vi "ke37xx Simple Switching Example.vi"() -> ()   [LabVIEW 2009]
doc: "Simple Switching Example \n\nThis sample demonstrates use of basic channel operations \nsupported by the Ke37XX. A channel list can be specified\non which various switch commands can be performed. After\neach switch operation, the current state of switch closures\nin the instrument is updated and displayed in the \"Channel \nStatus\" panel.\n\nUse of Pseudo Cards\n\nThis sample can be run using a mainframe that has no cards\npresent in the system slots (1 to 6). This is accomplished\nby use of the Ke37XX's native support for \"pseudo cards\".\nBy using pseudo cards, instrument commands may be sent to\nthe Ke37XX as if the cards were physically present. The \ninstrument responses will be simulated by the instrument itself.\nCombo boxes are provided for specifying which card should be\nsimulated in each slot."
uses:
  <instrlib>/Keithley 3706/Keithley 3700 Series.lvlib
panel:
  out "Close Channel List":string
  in  "Operation":T1(ring)
  in  "Channel List":string="1001:1005"
  in  "Slot 6 Pseudocard (6: 3740)":u16(ring)=6 items=["Empty", "3720", "3721", "3722", "3723", "3730", "3740"]
  in  "Slot 5 Pseudocard (5: 3730)":u16(ring)=5 items=["Empty", "3720", "3721", "3722", "3723", "3730", "3740"]
  in  "Slot 4 Pseudocard (4: 3723)":u16(ring)=4 items=["Empty", "3720", "3721", "3722", "3723", "3730", "3740"]
  in  "Slot 3 Pseudocard (3: 3722)":u16(ring)=3 items=["Empty", "3720", "3721", "3722", "3723", "3730", "3740"]
  in  "Slot 2 Pseudocard (2: 3721)":u16(ring)=2 items=["Empty", "3720", "3721", "3722", "3723", "3730", "3740"]
  in  "Slot 1 Pseudocard (1: 3720)":u16(ring)=1 items=["Empty", "3720", "3721", "3722", "3723", "3730", "3740"]
  in  "VISA Resource Name":refnum<visa-resource-name>="GPIB::6"
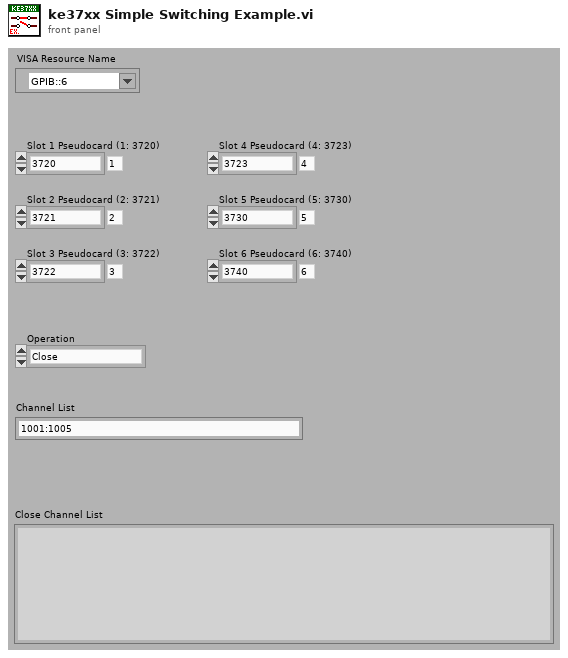
[diagram p1: front panel]
types:
  T1 = enum16{"Close", "Close Exclusive", "Close Slot Exclusive", "Open", "Open All"}
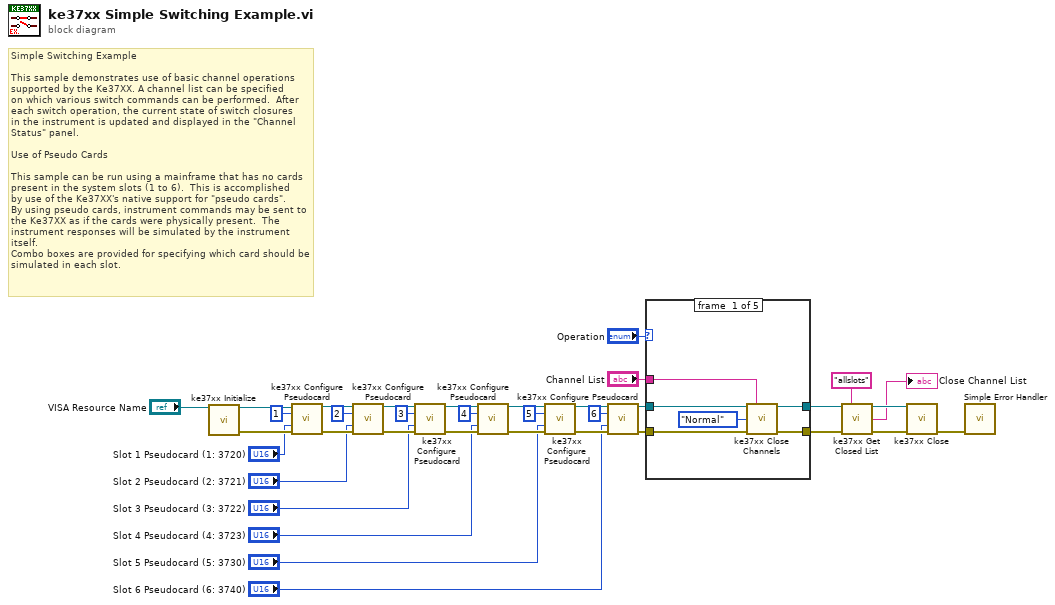
[diagram p0: block diagram]
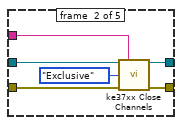
[diagram p2: hidden frame]
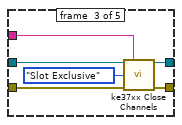
[diagram p3: hidden frame]
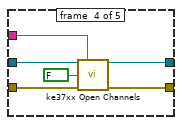
[diagram p4: hidden frame]
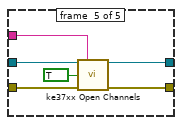
[diagram p5: hidden frame]
diagram:
  # "Simple Switching Example                              \n\nThis sample demonstrates use of basic channel operations \nsupported by the Ke37XX. A channel list can be specified\non which various switch commands can be performed.  After\neach switch operation, the current state of switch closures\nin the instrument is updated and displayed in the \"Channel \nStatus\" panel.\n\nUse of Pseudo Cards\n\nThis sample can be run using a mainframe that has no cards\npresent in the system slots (1 to 6).  This is accomplished\nby use of the Ke37XX's native support for \"pseudo cards\".\nBy using pseudo cards, instrument commands may be sent to\nthe Ke37XX as if the cards were physically present.  The \ninstrument responses will be simulated by the instrument itself.\nCombo boxes are provided for specifying which card should be\nsimulated in each slot."
  n1 = call <instrlib>:"ke37xx Initialize.vi"("VISA resource name"="VISA Resource Name") -> ("VISA resource name out"=w11:refnum<visa-resource-name>, "error out"=w36:errorcluster)  [unwired: 13 in]
  n2 = call <instrlib>:"ke37xx Configure Pseudocard.vi"("VISA Resource Name"=w11, "Slot Number (1)"=1, "Pseudocard Name (1: 3720)"="Slot 1 Pseudocard (1: 3720)", "error in (no error)"=w36) -> ("VISA Resource Name Out"=w27:refnum<visa-resource-name>, "error out"=w21:errorcluster)  [unwired: 10 in]
  n3 = call <instrlib>:"ke37xx Configure Pseudocard.vi"("VISA Resource Name"=w27, "Slot Number (1)"=2, "Pseudocard Name (1: 3720)"="Slot 2 Pseudocard (2: 3721)", "error in (no error)"=w21) -> ("VISA Resource Name Out"=w26:refnum<visa-resource-name>, "error out"=w20:errorcluster)  [unwired: 10 in]
  n4 = call <instrlib>:"ke37xx Configure Pseudocard.vi"("VISA Resource Name"=w26, "Slot Number (1)"=3, "Pseudocard Name (1: 3720)"="Slot 3 Pseudocard (3: 3722)", "error in (no error)"=w20) -> ("VISA Resource Name Out"=w25:refnum<visa-resource-name>, "error out"=w19:errorcluster)  [unwired: 10 in]
  n5 = call <instrlib>:"ke37xx Configure Pseudocard.vi"("VISA Resource Name"=w25, "Slot Number (1)"=4, "Pseudocard Name (1: 3720)"="Slot 4 Pseudocard (4: 3723)", "error in (no error)"=w19) -> ("VISA Resource Name Out"=w24:refnum<visa-resource-name>, "error out"=w18:errorcluster)  [unwired: 10 in]
  n6 = call <instrlib>:"ke37xx Configure Pseudocard.vi"("VISA Resource Name"=w24, "Slot Number (1)"=5, "Pseudocard Name (1: 3720)"="Slot 5 Pseudocard (5: 3730)", "error in (no error)"=w18) -> ("VISA Resource Name Out"=w23:refnum<visa-resource-name>, "error out"=w17:errorcluster)  [unwired: 10 in]
  n7 = call <instrlib>:"ke37xx Configure Pseudocard.vi"("VISA Resource Name"=w23, "Slot Number (1)"=6, "Pseudocard Name (1: 3720)"="Slot 6 Pseudocard (6: 3740)", "error in (no error)"=w17) -> ("VISA Resource Name Out"=w9:refnum<visa-resource-name>, "error out"=w8:errorcluster)  [unwired: 10 in]
  n8 = case shown="\"Close Slot Exclusive\"" "Operation" {
    tunnel: w9 -> [w42 w48 w54 w60 w66]
    tunnel: w8 -> [w41 w47 w53 w59 w65]
    tunnel: [w40 w46 w52 w58 w64] -> w7
    tunnel: [w39 w45 w51 w57 w63] -> w6
    tunnel: "Channel List" -> [w37 w43 w49 w56 w62]
    frame #0 {
      n9 = call <instrlib>:"ke37xx Close Channels.vi"("VISA Resource Name"=w42, "Channel List"=w37, "Mode (0: Normal)"=enum16{"Normal", "Exclusive", "Slot Exclusive"}."Normal", "error in (no error)"=w41) -> ("VISA Resource Name Out"=w40:refnum<visa-resource-name>, "error out"=w39:errorcluster)  [unwired: 10 in]
    }
    frame #1 {
      n10 = call <instrlib>:"ke37xx Close Channels.vi"("VISA Resource Name"=w48, "Channel List"=w43, "Mode (0: Normal)"=enum16{"Normal", "Exclusive", "Slot Exclusive"}."Exclusive", "error in (no error)"=w47) -> ("VISA Resource Name Out"=w46:refnum<visa-resource-name>, "error out"=w45:errorcluster)  [unwired: 10 in]
    }
    frame #2 {
      n11 = call <instrlib>:"ke37xx Close Channels.vi"("VISA Resource Name"=w54, "Channel List"=w49, "Mode (0: Normal)"=enum16{"Normal", "Exclusive", "Slot Exclusive"}."Slot Exclusive", "error in (no error)"=w53) -> ("VISA Resource Name Out"=w52:refnum<visa-resource-name>, "error out"=w51:errorcluster)  [unwired: 10 in]
    }
    frame #3 {
      n12 = call <instrlib>:"ke37xx Open Channels.vi"("VISA Resource Name"=w60, "Channel List"=w56, "Open All (False)"=FALSE, "error in (no error)"=w59) -> ("VISA Resource Name Out"=w58:refnum<visa-resource-name>, "error out"=w57:errorcluster)  [unwired: 10 in]
    }
    frame #4 {
      n13 = call <instrlib>:"ke37xx Open Channels.vi"("VISA Resource Name"=w66, "Channel List"=w62, "Open All (False)"=TRUE, "error in (no error)"=w65) -> ("VISA Resource Name Out"=w64:refnum<visa-resource-name>, "error out"=w63:errorcluster)  [unwired: 10 in]
    }
  }
  n14 = call <instrlib>:"ke37xx Get Closed List.vi"("VISA Resource Name"=w7, "Channel List"="allslots", "error in (no error)"=w6) -> ("VISA Resource Name Out"=w5:refnum<visa-resource-name>, "Closed List"=→"Close Channel List":string, "error out"=w4:errorcluster)  [unwired: 10 in]
  n15 = call <instrlib>:"ke37xx Close.vi"("VISA resource name"=w5, "error in (no error)"=w4) -> ("error out"=w34:errorcluster)  [unwired: 13 in]
  n16 = call <vilib>:"Simple Error Handler.vi"("error in (no error)"=w34) -> ()  [unwired: 1 in, 8 out]
